vi "MListbox Delete Selected.vi"(8 "error in (no error)":errorcluster, 11 "Multicolumn ListBox in":refnum<class "Multicolumn ListBox.lvclass">) -> (0 "error out":errorcluster, 3 "Multicolumn ListBox out":refnum<class "Multicolumn ListBox.lvclass">)   [LabVIEW 2018, in "Multicolumn ListBox.lvclass"]
uses:
  Multicolumn ListBox.lvclass
  Multicolumn ListBox.lvclass/Multicolumn ListBox.ctl
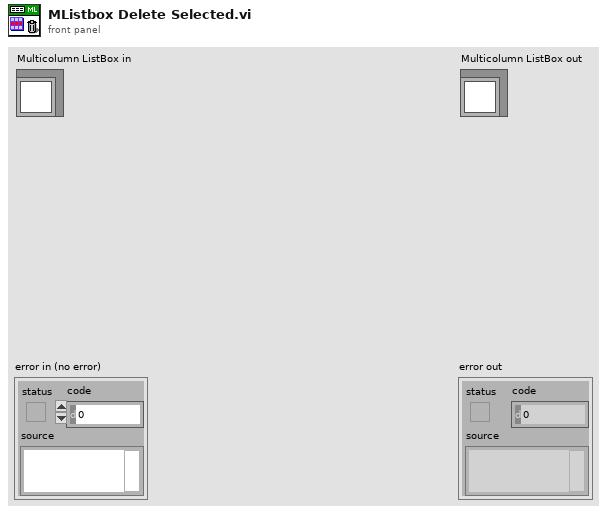
[diagram p1: front panel]
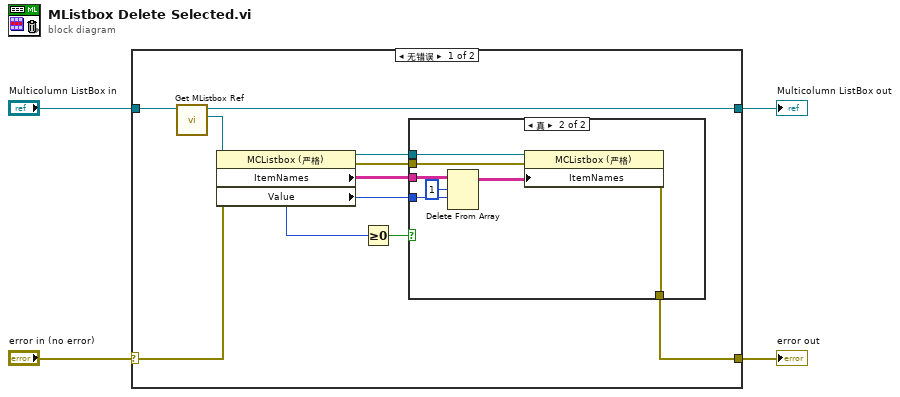
[diagram p0: block diagram]
diagram:
  n1 = case shown="无错误" "error in (no error)" {
    selector: "error in (no error)" -> [w9 w24]
    tunnel: [w8 w24] -> w3
    tunnel: [w13 w23] -> w1
    tunnel: "Multicolumn ListBox in" -> [w14 w23]
    frame No Error {
      n2 = call "Get MListbox Ref.vi"("Multicolumn ListBox in"=w14) -> ("MListbox Ref"=w12:refnum<vi>, "Multicolumn ListBox out"=w13:refnum<class "Multicolumn ListBox.lvclass">)  [unwired: 8 in, 1 out]
      n3 = property class="MCListbox (严格)"(reference=w12, error in=w9) -> (reference out=w11:refnum<vi>, error out=w10:errorcluster, "ItemNames"=w6:string[][], "Value"=w5:i32)
      n4 = Greater Or Equal To 0?(x=w5) -> (x >= 0?=w7:bool)
      n5 = case shown="真" w7 {
        tunnel: w11 -> [_ w22]
        tunnel: w10 -> [w15 w21]
        tunnel: [w15 w20] -> w8
        tunnel: w6 -> [_ w19]
        tunnel: w5 -> [_ w18]
        frame False {
        }
        frame True {
          n6 = Delete From Array ("删除数组元素")(array=w19, length=1, index (row)=w18) -> (array with subset deleted=w16:string[][])  [unwired: 1 in, 1 out]
          n7 = property class="MCListbox (严格)"(reference=w22, error in=w21, "ItemNames"=w16) -> (error out=w20:errorcluster)  [unwired: 1 out]
        }
      }
    }
    frame Error {
    }
  }
  "error out" <- w3
  "Multicolumn ListBox out" <- w1
